vi "Configure Multi Eval Meas Limit FERR.vi"(6 "Limit Value (0.1)":dbl=0.1 format="%^.3e", 7 "Limit Check Enabled (Off)":i32(ring) items=["Off", "On", "Value"], 8 "error in (no error)":errorcluster, 9 "Modulation (Pi/2-BPSK)":i32(ring) items=["Pi/2-BPSK", "QPSK", "16-QAM", "64-QAM", "256-QAM"], 10 "Instance (1)":T1=1, 11 "VISA resource name":refnum<visa-resource-name>) -> (0 "error out":errorcluster, 3 "VISA resource name out":refnum<visa-resource-name>)   [LabVIEW 2015, in "Rohde&Schwarz CMXP NR FR2 Measurement.lvlib"]
doc: "Defines an upper limit for the carrier frequency error.\n\nAttributes:\nRSCMXPNRFR2M_ATTR_MULTI_EVAL_MEASUREMENT_LIMIT_PHBPSK_FERR\nRSCMXPNRFR2M_ATTR_MULTI_EVAL_MEASUREMENT_LIMIT_QPSK_FERR\nRSCMXPNRFR2M_ATTR_MULTI_EVAL_MEASUREMENT_LIMIT_QAM16_FERR\nRSCMXPNRFR2M_ATTR_MULTI_EVAL_MEASUREMENT_LIMIT_QAM64_FERR\nRSCMXPNRFR2M_ATTR_MULTI_EVAL_MEASUREMENT_LIMIT_QAM256_FERR\n\nRemote-control commands:\nCONFigure:NRMMw:MEAS<i>:MEValuation:LIMit:PHBPsk:FERRor\nCONFigure:NRMMw:MEAS<i>:MEValuation:LIMit:QPSK:FERRor\nCONFigure:NRMMw:MEAS<i>:MEValuation:LIMit:QAM<order>:FERRor"
uses:
  <instrlib>/Rohde&Schwarz CMXP NR FR2 Measurement/Rohde&Schwarz CMXP NR FR2 Measurement.lvlib
  <instrlib>/Rohde&Schwarz CMXP NR FR2 Measurement/Private/_Instance.ctl
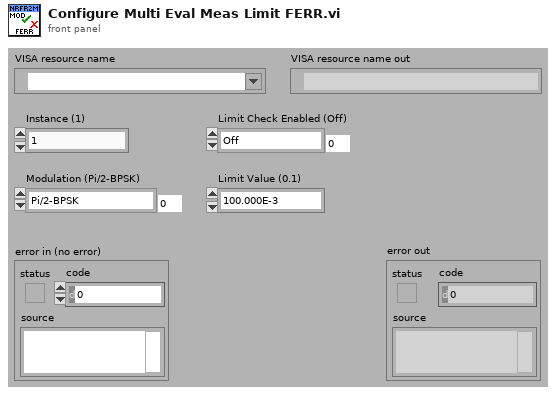
[diagram p1: front panel]
types:
  T1 = typedef "Rohde&Schwarz CMXP NR FR2 Measurement.lvlib/_Instance.ctl" = i32
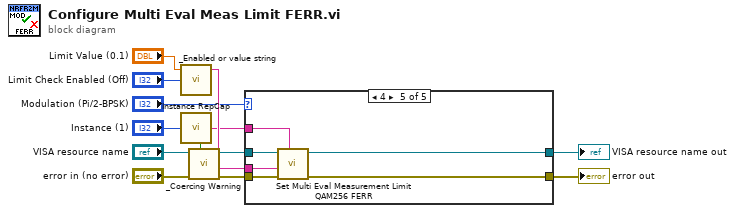
[diagram p0: block diagram]
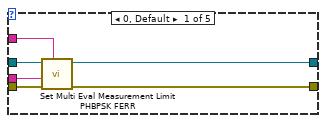
[diagram p2: hidden frame]
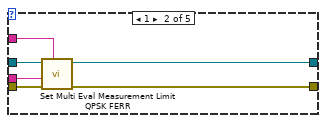
[diagram p3: hidden frame]
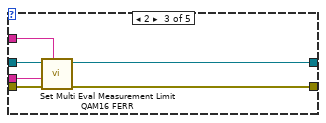
[diagram p4: hidden frame]
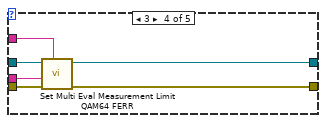
[diagram p5: hidden frame]
diagram:
  n1 = call <instrlib>:"_Enabled or value string.vi"("Enabled or Value"="Limit Check Enabled (Off)", "Value"="Limit Value (0.1)") -> ("Resulting String"=w6:string)  [unwired: 3 in]
  n2 = call <instrlib>:"Instance RepCap.vi"("Instance In"="Instance (1)") -> ("In Range?"=w10:bool, "RepCap Identifier Out"=w5:string)  [unwired: 1 in]
  n3 = call <instrlib>:"_Coercing Warning.vi"("In Range?"=w10, "error in (no error)"="error in (no error)", "VISA resource name"="VISA resource name") -> ("error out"=w8:errorcluster, "VISA resource name out"=w7:refnum<visa-resource-name>)  [unwired: 7 in]
  n4 = case shown="4" "Modulation (Pi/2-BPSK)" {
    tunnel: w8 -> [w19 w25 w31 w37 w43]
    tunnel: w7 -> [w18 w24 w30 w36 w42]
    tunnel: w6 -> [w14 w20 w26 w32 w38]
    tunnel: w5 -> [w17 w23 w29 w35 w41]
    tunnel: [w16 w22 w28 w34 w40] -> w3
    tunnel: [w15 w21 w27 w33 w39] -> w2
    frame 0, Default {
      n5 = call "Set Multi Eval Measurement Limit PHBPSK FERR"("Repeated Capabilities"=w17, "error in (no error)"=w19, "Multi Eval Measurement Limit PHBPSK FERR ()"=w14, "instrument handle"=w18) -> ("error out"=w16:errorcluster, "instrument handle out"=w15:refnum<visa-resource-name>)  [unwired: 6 in]
    }
    frame 1 {
      n6 = call "Set Multi Eval Measurement Limit QPSK FERR"("Repeated Capabilities"=w23, "error in (no error)"=w25, "Multi Eval Measurement Limit QPSK FERR ()"=w20, "instrument handle"=w24) -> ("error out"=w22:errorcluster, "instrument handle out"=w21:refnum<visa-resource-name>)  [unwired: 6 in]
    }
    frame 2 {
      n7 = call "Set Multi Eval Measurement Limit QAM16 FERR"("Repeated Capabilities"=w29, "error in (no error)"=w31, "Multi Eval Measurement Limit QAM16 FERR ()"=w26, "instrument handle"=w30) -> ("error out"=w28:errorcluster, "instrument handle out"=w27:refnum<visa-resource-name>)  [unwired: 6 in]
    }
    frame 3 {
      n8 = call "Set Multi Eval Measurement Limit QAM64 FERR"("Repeated Capabilities"=w35, "error in (no error)"=w37, "Multi Eval Measurement Limit QAM64 FERR ()"=w32, "instrument handle"=w36) -> ("error out"=w34:errorcluster, "instrument handle out"=w33:refnum<visa-resource-name>)  [unwired: 6 in]
    }
    frame 4 {
      n9 = call "Set Multi Eval Measurement Limit QAM256 FERR"("Repeated Capabilities"=w41, "error in (no error)"=w43, "Multi Eval Measurement Limit QAM256 FERR ()"=w38, "instrument handle"=w42) -> ("error out"=w40:errorcluster, "instrument handle out"=w39:refnum<visa-resource-name>)  [unwired: 6 in]
    }
  }
  "error out" <- w3
  "VISA resource name out" <- w2
